vi "SearchFrameStartProcesses.vi"(8 "error in (no error)":errorcluster, 11 "AppContextIn":T1={"VIRefToProcessTemplate"=refnum, "VIRefToThisVI"=refnum, "ProcessesList"=[], "VIRefToEnumProcess"=refnum, "VIRefTogetProcessViPath"=refnum, "ProcessManagement"={"EnumProcessState"=enum."Create process", "ProcessName"="", "PathToProcess"=path ""}, "VIRefToSetup"=refnum, "VIRefToStartProcess"=refnum, "ProcessConfig"={"File Path Control"=path "", "Timeout"=0.0, "viInitString"="", "State"=enum."Closed"}}) -> (0 "error out":errorcluster, 2 "FlatSequenceFrame out":refnum<vi>, 3 "AppContextOut":T1={"VIRefToProcessTemplate"=refnum, "VIRefToThisVI"=refnum, "ProcessesList"=[], "VIRefToEnumProcess"=refnum, "VIRefTogetProcessViPath"=refnum, "ProcessManagement"={"EnumProcessState"=enum."Create process", "ProcessName"="", "PathToProcess"=path ""}, "VIRefToSetup"=refnum, "VIRefToStartProcess"=refnum, "ProcessConfig"={"File Path Control"=path "", "Timeout"=0.0, "viInitString"="", "State"=enum."Closed"}})   [LabVIEW 2011]
uses:
  Ctl/AppContext.ctl
  Ctl/EnumProcessState.ctl
  050 - CONFIG/20 - ExternalProcesses/paramsExternalProcesses.ctl
  <vilib>/Utility/traverseref.llb/TRef TravTarget.ctl
  <vilib>/Utility/traverseref.llb/VI Scripting - Traverse.lvlib
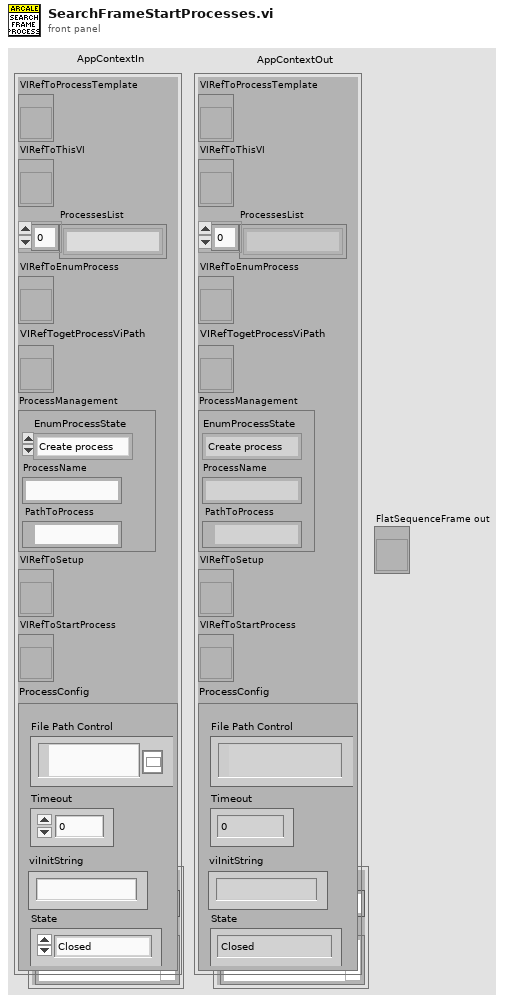
[diagram p1: front panel]
types:
  T1 = typedef "AppContext.ctl" = cluster{"VIRefToProcessTemplate":refnum<vi>, "VIRefToThisVI":refnum<vi>, "ProcessesList":string[], "VIRefToEnumProcess":refnum<vi>, "VIRefTogetProcessViPath":refnum<vi>, "ProcessManagement":cluster{"EnumProcessState":T2, "ProcessName":string, "PathToProcess":path}, "VIRefToSetup":refnum<vi>, "VIRefToStartProcess":refnum<vi>, "ProcessConfig":T3}
  T2 = typedef "EnumProcessState.ctl" = enum16{"Create process", "Delete process"}
  T3 = typedef "paramsExternalProcesses.ctl" = cluster{"File Path Control":path, "Timeout":dbl, "viInitString":string, "State":enum32{"Invalid", "Standard", "Closed", "Hidden", "Minimized", "Maximized"}}
  T4 = typedef "TRef TravTarget.ctl" = enum16{"FP", "BD", "Other"}
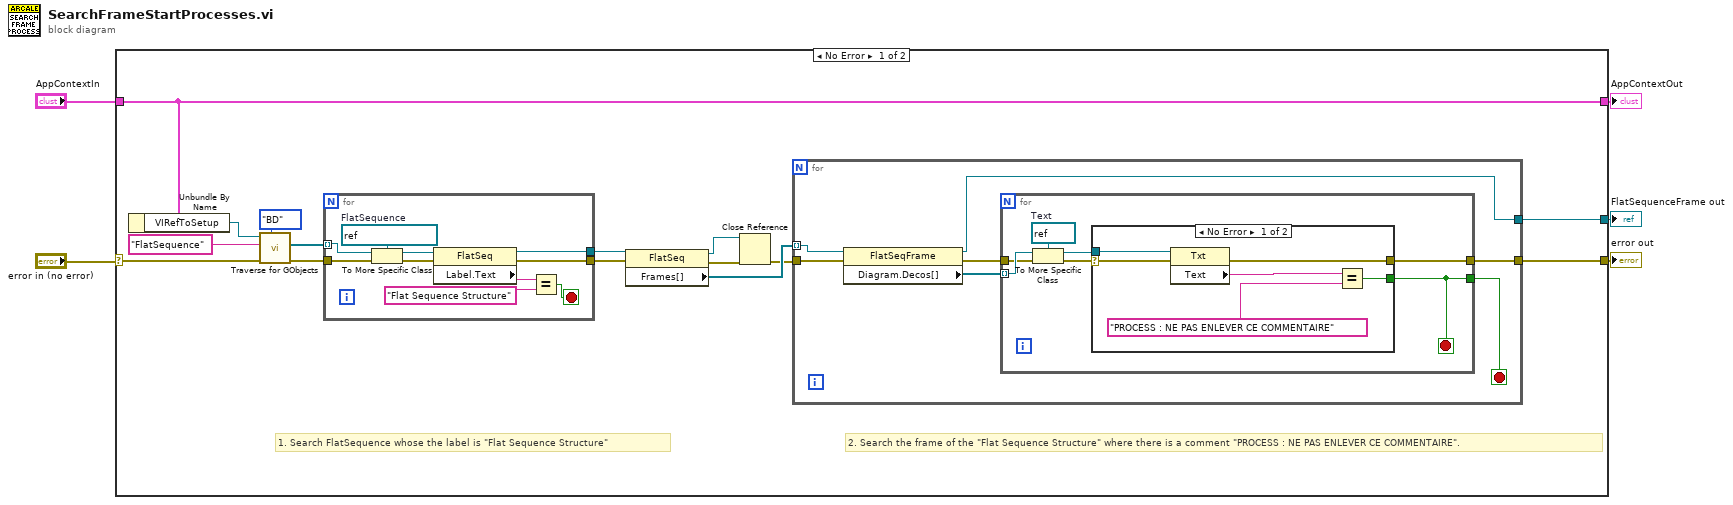
[diagram p0: block diagram]
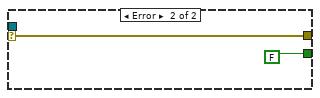
[diagram p2: hidden frame]
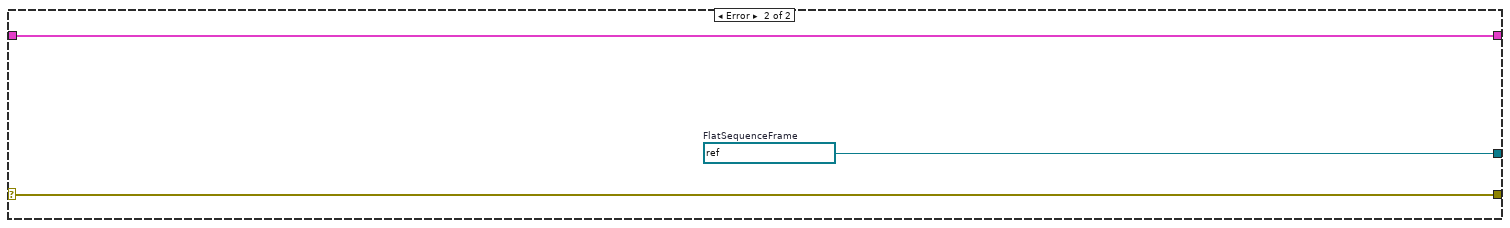
[diagram p3: hidden frame]
diagram:
  n1 = case shown="No Error" "error in (no error)" {
    selector: "error in (no error)" -> [w14 w54]
    tunnel: [w20 w54] -> w5
    tunnel: [w19 w55] -> w4
    tunnel: "AppContextIn" -> [w12 w53]
    tunnel: [w12 w53] -> w1
    frame No Error {
      # "2. Search the frame of the \"Flat Sequence Structure\" where there is a comment \"PROCESS : NE PAS ENLEVER CE COMMENTAIRE\"."
      # "1. Search FlatSequence whose the label is \"Flat Sequence Structure\""
      n2 = Unbundle By Name(w12) -> ("VIRefToSetup"=w15:refnum<vi>)
      n3 = call <vilib>:"Traverse for GObjects.vi"("Traverse Target"=TRef_TravTarget."BD", "error in (no error)"=w14, "Class Name"="FlatSequence", "VI Refnum"=w15) -> ("error out"=w11:errorcluster, "References"=w17:refnum<vi>[])  [unwired: 4 in, 2 out]
      n4 = for {
        tunnel: w17 -> [w28] mode=indexing
        tunnel: w11 -> [w29]
        tunnel: [w23] -> w10
        tunnel: [w21] -> w9
        stop <- w24 stop-if-true
        w30 = refnum<vi> refnum  # FlatSequence
        n5 = To More Specific Class(target class=w30, reference=w28, error in=w29) -> (specific class reference=w27:refnum<vi>, error out=w22:errorcluster)
        n6 = property class="FlatSeq"(reference=w27, error in=w22) -> (reference out=w23:refnum<vi>, error out=w21:errorcluster, "Label.Text"=w26:string)
        n7 = Equal?(x=w26, y="Flat Sequence Structure") -> (x = y?=w24:bool)
      }
      n8 = property class="FlatSeq"(reference=w10, error in=w9) -> (reference out=w6:refnum<vi>, error out=w7:errorcluster, "Frames[]"=w13:refnum<vi>[])
      n9 = Close Reference(reference=w6, error in (no error)=w7) -> (error out=w8:errorcluster)
      n10 = for {
        tunnel: w13 -> [w37] mode=indexing
        tunnel: [w35] -> w19
        tunnel: w8 -> [w33]
        tunnel: [w31] -> w20
        stop <- w34 stop-if-true
        n11 = property class="FlatSeqFrame"(reference=w37, error in=w33) -> (reference out=w35:refnum<vi>, error out=w32:errorcluster, "Diagram.Decos[]"=w36:refnum<vi>[])
        n12 = for {
          tunnel: w36 -> [w44] mode=indexing
          tunnel: [w41] -> w34
          tunnel: w32 -> [w40]
          tunnel: [w38] -> w31
          stop <- w41 stop-if-true
          w43 = refnum<vi> refnum  # Text
          n13 = To More Specific Class(target class=w43, reference=w44, error in=w40) -> (specific class reference=w42:refnum<vi>, error out=w39:errorcluster)
          n14 = case shown="No Error" w39 {
            selector: w39 -> [w47 w51]
            tunnel: w42 -> [w50 _]
            tunnel: [w48 FALSE] -> w41
            tunnel: [w46 w51] -> w38
            frame No Error {
              n15 = property class="Txt"(reference=w50, error in=w47) -> (error out=w46:errorcluster, "Text"=w49:string)  [unwired: 1 out]
              n16 = Equal?(x=w49, y="PROCESS : NE PAS ENLEVER CE COMMENTAIRE") -> (x = y?=w48:bool)
            }
            frame Error {
            }
          }
        }
      }
    }
    frame Error {
      w55 = refnum<vi> refnum  # FlatSequenceFrame
    }
  }
  "error out" <- w5
  "FlatSequenceFrame out" <- w4
  "AppContextOut" <- w1
